vi "annotate image.vi"(0 "Detection string":string, 4 "Color":u32, 6 "CamConfigArray":T3, 7 "rescale":bool, 8 "Image Dst":T1, 10 "Font, Size & Style":T4={"Desired Font (Application)"=enum."User-specified Font", "[User-specified Font]"={"Font Name"="Arial", "Size"=20, "Strikeout?"=FALSE, "Italic?"=FALSE, "Underline?"=TRUE, "Outline?"=FALSE, "Shadow?"=FALSE, "Bold?"=TRUE, "Rotation Angle"=0.0}, "Horizontal Alignment"=1, "Vertical Alignment"=0}, 11 "Image in":T1) -> (1 "Maximal Value":sgl, 3 "Image Dst Out":T1)   [LabVIEW 2013]
uses:
  <vilib>/vision/Image Controls.llb/IMAQ Image.ctl
  <vilib>/userdefined/High Color/IMAQdx.ctl
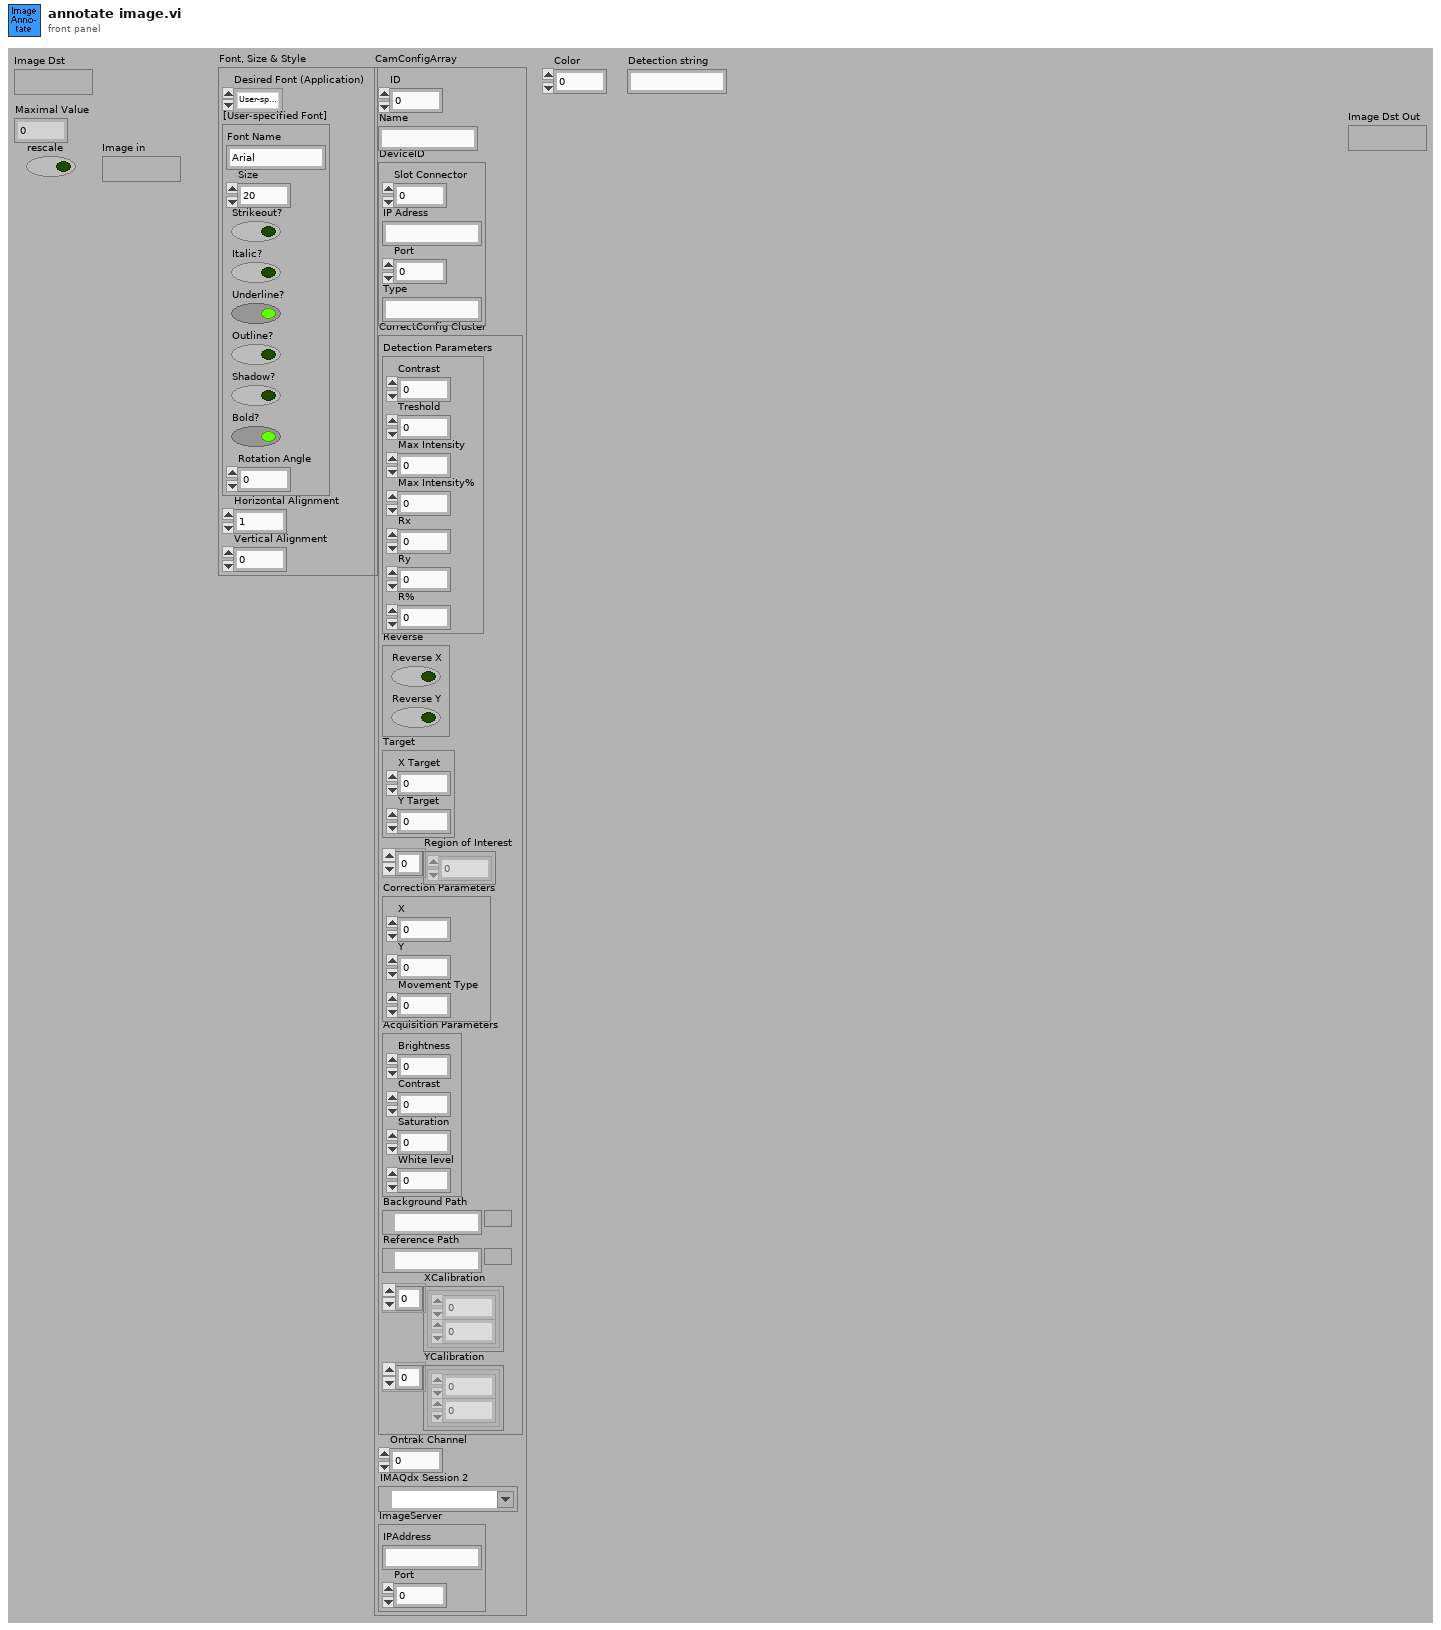
[diagram p1: front panel]
types:
  T1 = typedef "IMAQ Image.ctl" = refnum<image>
  T2 = typedef "IMAQdx.ctl" = refnum<k21>
  T3 = cluster{"ID":dbl, "Name":string, "DeviceID":cluster{"Slot Connector":i32, "IP Adress":string, "Port":i32, "Type":string}, "CorrectConfig Cluster":cluster{"Detection Parameters":cluster{"Contrast":i32, "Treshold":u8, "Max Intensity":i32, "Max Intensity%":u8, "Rx":i32, "Ry":i32, "R%":sgl}, "Reverse":cluster{"Reverse X":bool, "Reverse Y":bool}, "Target":cluster{"X Target":sgl, "Y Target":sgl}, "Region of Interest":i32[], "Correction Parameters":cluster{"X":sgl, "Y":sgl, "Movement Type":u16}, "Acquisition Parameters":cluster{"Brightness":dbl, "Contrast":dbl, "Saturation":dbl, "White level":dbl}, "Background Path":path, "Reference Path":path, "XCalibration":cluster{dbl, dbl}[], "YCalibration":cluster{dbl, dbl}[]}, "Ontrak Channel":i16, "IMAQdx Session 2":T2, "ImageServer":cluster{"IPAddress":string, "Port":i32}}
  T4 = cluster{"Desired Font (Application)":enum16{"User-specified Font", "Application Font", "System Font", "Dialog Font"}, "[User-specified Font]":cluster{"Font Name":string, "Size":i16, "Strikeout?":bool, "Italic?":bool, "Underline?":bool, "Outline?":bool, "Shadow?":bool, "Bold?":bool, "Rotation Angle":dbl}, "Horizontal Alignment":i16, "Vertical Alignment":i16}
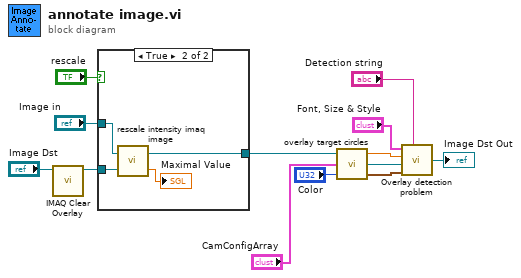
[diagram p0: block diagram]
diagram:
  n1 = call "IMAQ Clear Overlay"("Image"="Image Dst") -> ("Image Out"=w1:T1)  [unwired: 9 in, 1 out]
  n2 = case shown="True" "rescale" {
    tunnel: [w14 w18] -> w5
    tunnel: "Image in" -> [w14 w17]
    tunnel: w1 -> [_ w16]
    frame False {
    }
    frame True {
      n3 = call "rescale intensity imaq image.vi"("Image Dst"=w16, "Image in"=w17) -> ("Maximal Value"=→"Maximal Value":sgl, "Image Dst Out"=w18:T1)
    }
  }
  n4 = call "overlay target circles.vi"("Color"="Color", "CamConfigArray"="CamConfigArray", "Image Dst Out"=w5) -> ("Cluster"=w8:cluster{"X Target":sgl, dbl}, "Image Out"=w10:T1, "Numeric"=w6:dbl)
  n5 = call "Overlay detection problem.vi"("Font, Size & Style"="Font, Size & Style", "Font Size"=w6, "Image In"=w10, "Origin"=w8, "Detection string"="Detection string") -> ("Image Out"=→"Image Dst Out":T1)
